vi "CRYTSR Time Envelope.vi"(8 "Fs":dbl=44100.0, 9 "FMax":dbl=2000.0, 10 "FMin":dbl=1000.0, 11 "Response":dbl[](array[numeric])=[0.0, 0.0, 0.0, 0.0, 0.0, 1.0, 0.0, 0.0, 0.0, 0.0, 0.0] format="%.2f") -> (1 "Magn":dbl[](array[numeric])=[0.12716412468699562, 0.0, 0.21211070832577886, 0.0, 0.6365878141136418, 1.0, 0.6365878141136421, 0.0, 0.21211070832577902, 0.0, 0.12716412468699528] format="%.2f", 2 "Imag":dbl[](array[numeric])=[-0.12716412468699562, 0.0, -0.21211070832577886, 0.0, -0.6365878141136418, 0.0, 0.6365878141136421, 0.0, 0.21211070832577902, 0.0, 0.12716412468699528] format="%.2f", 3 "Real":dbl[](array[numeric])=[0.0, 0.0, 0.0, 0.0, 0.0, 1.0, 0.0, 0.0, 0.0, 0.0, 0.0] format="%.2f")   [LabVIEW 2013]
uses:
  <vilib>/Analysis/2dsp.llb/Decimate (single shot, DBL).vi
  <vilib>/Analysis/NI_AALBase.lvlib
  <vilib>/Analysis/NI_AALPro.lvlib
  <vilib>/Analysis/2dsp.llb/1D Convolution (DBL).vi
  <vilib>/Analysis/4window.llb/Hanning Window (DBL).vi
  <vilib>/Analysis/4window.llb/Flat Top Window (DBL).vi
panel:
  out "Waveform Graph":waveform(dbl)(graph)
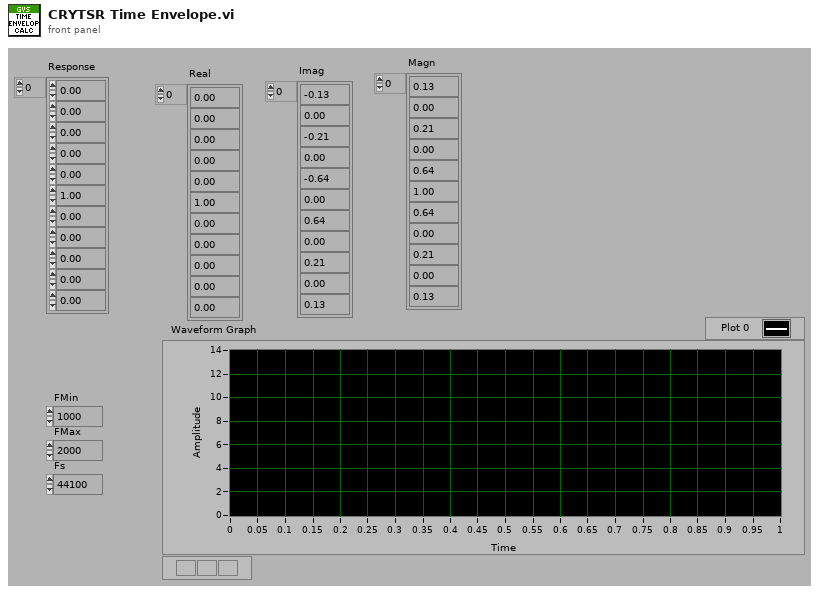
[diagram p1: front panel]
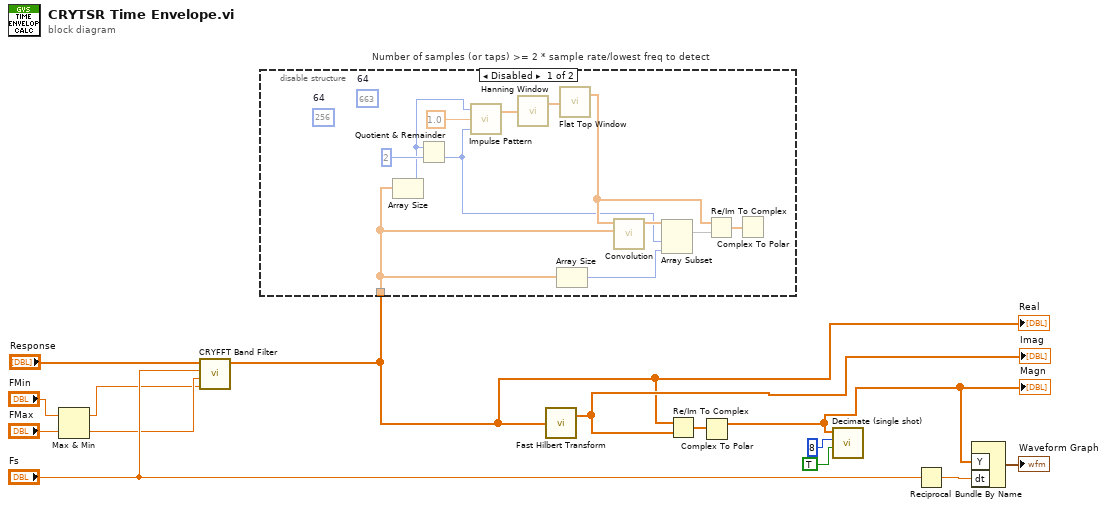
[diagram p0: block diagram]
diagram:
  # "Number of samples (or taps) >= 2 * sample rate/lowest freq to detect"
  n1 = Max & Min(x="FMin", y="FMax") -> (max(x,y)=w3:dbl, min(x,y)=w4:dbl)
  n2 = call "CRYFFT Band Filter.vi"("High Freq"=w3, "Low Freq"=w4, "Fs"="Fs", "Signal In"="Response") -> ("Signal out"=w9:dbl[])  [unwired: 7 in]
  "Real" <- w9
  n3 = disable-structure shown="Disabled" {
    disable-tunnel: w9 -> [w15 _]
    frame Disabled {
      (unwired) 256  # 64
      (unwired) 663  # 64
      n4 = Array Size(array=w15) -> (size(s)=w16:i32)
      n5 = Quotient & Remainder(x=w16, y=2) -> (floor(x/y)=w17:i32)  [unwired: 1 out]
      n6 = call <vilib>:"Impulse Pattern.vi"("delay"=w17, "amplitude"=1.0, "samples"=w16) -> ("Impulse Pattern"=w19:dbl[])  [unwired: 1 out]
      n7 = call-poly <vilib>:"Hanning Window.vi"("X"=w19) -> ("Windowed X"=w21:dbl[])  [unwired: 1 out]
      n8 = Array Size(array=w15) -> (size(s)=w20:i32)
      n9 = call-poly <vilib>:"Flat Top Window.vi"("X"=w21) -> ("Windowed X"=w18:dbl[])  [unwired: 1 out]
      n10 = call-poly <vilib>:"Convolution.vi"("Y"=w15, "X"=w18) -> ("X * Y"=w23:dbl[])  [unwired: 1 in, 8 out]
      n11 = Array Subset(array=w23, index=w17, length=w20) -> (w22:dbl[])
      n12 = Re/Im To Complex(1:w22, 2:w18) -> (0:w25:cdb[])
      n13 = Complex To Polar(r * e^(i*theta)=w25) -> ()  [unwired: 2 out]
    }
    frame Enabled {
    }
  }
  n14 = call <vilib>:"Fast Hilbert Transform.vi"("X"=w9) -> ("Hilbert{X}"=w10:dbl[])  [unwired: 1 out]
  "Imag" <- w10
  n15 = Re/Im To Complex(1:w10, 2:w9) -> (0:w2:cdb[])
  n16 = Complex To Polar(r * e^(i*theta)=w2) -> (r=w1:dbl[])  [unwired: 1 out]
  "Magn" <- w1
  n17 = call-poly <vilib>:"Decimate (single shot).vi"("averaging"=TRUE, "decimating factor"=8, "X"=w1) -> ()  [unwired: 9 out]
  n18 = Reciprocal(x="Fs") -> (1/x=w14:dbl)
  n19 = Bundle By Name("Y"=w1, "dt"=w14) -> (→"Waveform Graph":waveform(dbl))  [unwired: 1 in]
